vi "Check Admin Rights.vi"(3 "Error In":errorcluster) -> (8 "Admin?":bool, 10 "Error Out":errorcluster)   [LabVIEW 2017]
doc: "This VI determines if the current instance of LabVIEW is running with adminstrator privileges."
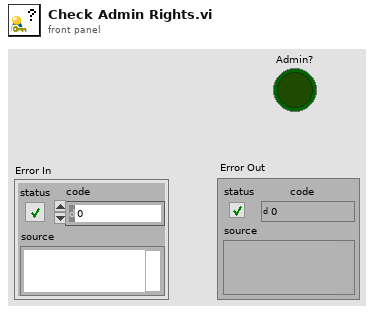
[diagram p1: front panel]
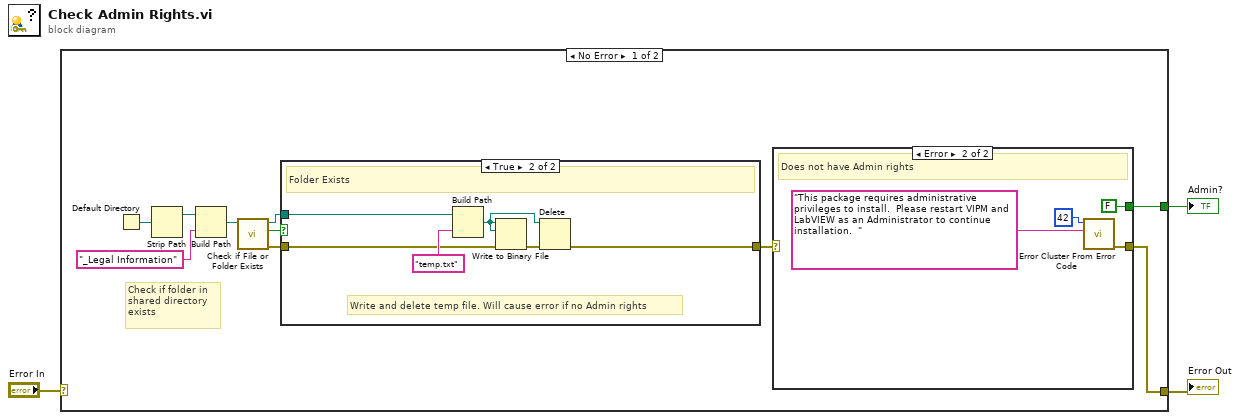
[diagram p0: block diagram]
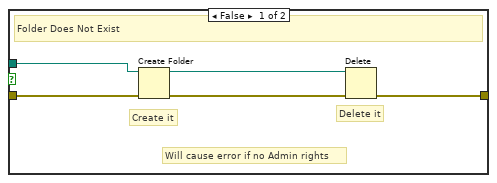
[diagram p2: hidden frame]
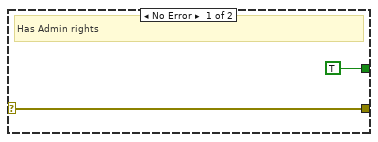
[diagram p3: hidden frame]
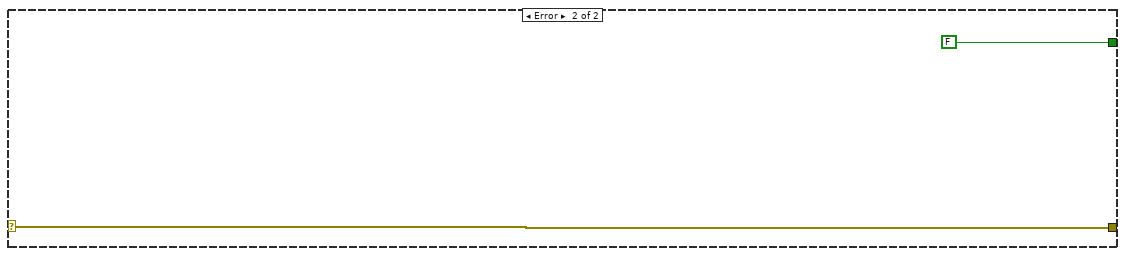
[diagram p4: hidden frame]
diagram:
  n1 = case shown="No Error" "Error In" {
    selector: "Error In" -> [_ w32]
    tunnel: [w13 w32] -> w2
    tunnel: [w6 FALSE] -> w1
    frame No Error {
      # "Check if folder in\nshared directory\nexists"
      n2 = Default Directory() -> (w10:path)
      n3 = Strip Path(path=w10) -> (stripped path=w9:path)  [unwired: 1 out]
      n4 = Build Path(base path=w9, name or relative path="_Legal Information" ("string")) -> (appended path=w8:path)
      n5 = call <vilib>:"Check if File or Folder Exists.vi"("path"=w8) -> ("error out"=w11:errorcluster, "file or folder exists?"=w5:bool, "dup path"=w12:path)  [unwired: 8 in]
      n6 = case shown="True" w5 {
        tunnel: w12 -> [w18 w21]
        tunnel: w11 -> [w17 w20]
        tunnel: [w15 w19] -> w4
        frame False {
          # "Will cause error if no Admin rights"
          # "Delete it"
          # "Create it"
          # "Folder Does Not Exist"
          n7 = Create Folder(path (use dialog)=w18, error in=w17) -> (created path=w14:path, error out=w16:errorcluster)  [unwired: 1 in, 1 out]
          n8 = Delete(path (use dialog)=w14, error in=w16) -> (error out=w15:errorcluster)  [unwired: 3 in, 2 out]
        }
        frame True {
          # "Write and delete temp file. Will cause error if no Admin rights"
          # "Folder Exists"
          n9 = Build Path(base path=w21, name or relative path="temp.txt" ("string")) -> (appended path=w24:path)
          n10 = Write to Binary File(file (use dialog)=w24, data=w24, error in=w20) -> (error out=w23:errorcluster)  [unwired: 3 in, 2 out]
          n11 = Delete(path (use dialog)=w24, error in=w23) -> (error out=w19:errorcluster)  [unwired: 3 in, 2 out]
        }
      }
      n12 = case shown="Error" w4 {
        selector: w4 -> [w26 _]
        tunnel: [w26 w28] -> w13
        tunnel: [TRUE FALSE] -> w6
        frame No Error {
          # "Has Admin rights"
        }
        frame Error {
          # "Does not have Admin rights"
          n13 = call <vilib>:"Error Cluster From Error Code.vi"("error message (\"\")"="This package requires administrative privileges to install.  Please restart VIPM and LabVIEW as an Administrator to continue installation.  " ("error message (\"\")"), "error code (0)"=42) -> ("error out"=w28:errorcluster)  [unwired: 7 in]
        }
      }
    }
    frame Error {
    }
  }
  "Error Out" <- w2
  "Admin?" <- w1
